vi "Check for Contained Data Type.vi"(4 "Type Specific Details":T1, 6 "Check VI Refnum Connector Pane? (F)":bool, 8 "error in (no error)":errorcluster, 10 "Data Type to Find":T2, 11 "Data Type":variant) -> (0 "error out":errorcluster, 2 "Contains Data Type to Find?":bool, 3 "dup Data Type":variant)   [LabVIEW 2020]
doc: "This VI is deprecated. Use the following VI instead:\n\nvi.lib\\Utility\\Data Type\\Check for Contained Data Type.vi\n\nThis VI checks the \"Data Type\" input to see if it contains any sub-types that are of type \"Data Type to Find\". If so, the \"Contains Data Type to Find?\" output is True.\n\nFor example, if \"Data Type\" is a cluster containing many items, including a Boolean data type, if \"Data Type to Find\" is \"Boolean\", the VI will return a \"Contains Data Type to Find?\" value of True."
uses:
  <vilib>/Utility/VariantDataType/Type.ctl
  <vilib>/Utility/VariantDataType/Type Specific Details.ctl
  <vilib>/Utility/VariantDataType/VariantType.lvlib
panel:
  # "This VI is deprecated. Use the following VI instead:\n\nvi.lib\\Utility\\Data Type\\Check for Contained Data Type.vi"
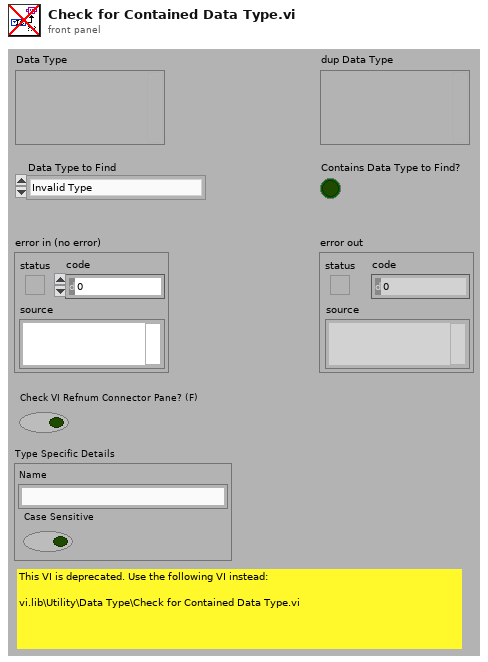
[diagram p1: front panel]
types:
  T1 = typedef "Type Specific Details.ctl" = cluster{"Name":string, "Case Sensitive":bool}
  T2 = typedef "VariantType.lvlib/Type.ctl" = enum8{"Invalid Type", "Void", "I8", "I16", "I32", "I64", "U8", "U16", "U32", "U64", "Single Float", "Double Float", "Extended Float", "Single Complex", "Double Complex", "Extended Complex", "Enum U8", "Enum U16", "Enum U32", "Enum U64", "Single Float With Unit", "Double Float With Unit", "Extended Float With Unit", "Single Complex with Unit", "Double Complex with Unit", "Extended Complex with Unit", "Boolean", "String", "Path", "Picture", "Tag", "Array", "Cluster", "Variant", "LV Variant", "Waveform", "Timestamp", "Digital Waveform", "Digital Data", "ExpressData", "Refnum", "External Data", "VI", "Poly VI", "LabVIEW Class Instance", "Fixed Point"}
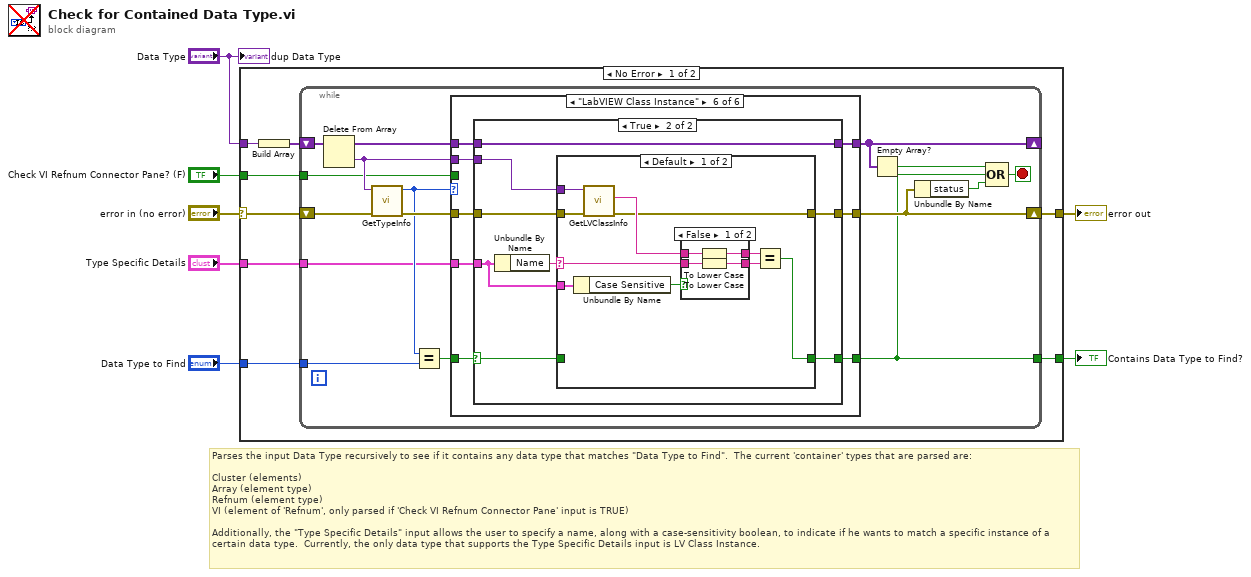
[diagram p0: block diagram]
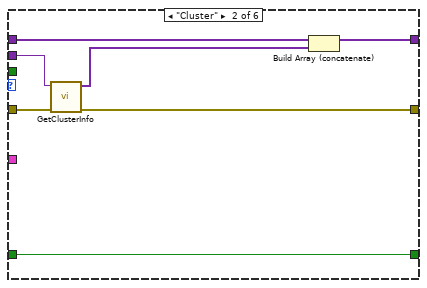
[diagram p3: hidden frame]
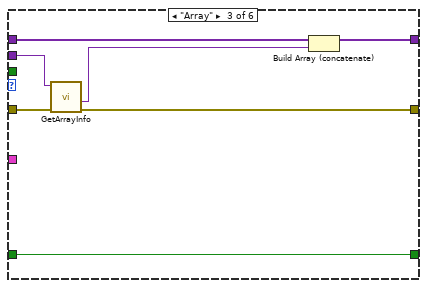
[diagram p4: hidden frame]
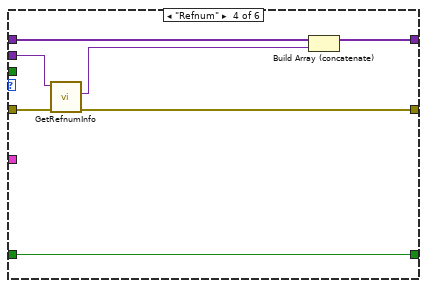
[diagram p5: hidden frame]
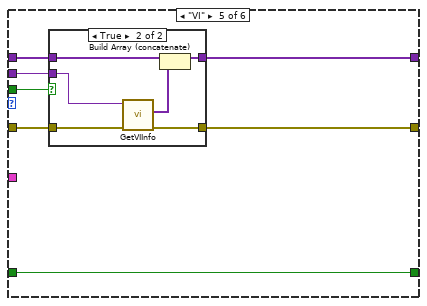
[diagram p6: hidden frame]
diagram:
  # "Parses the input Data Type recursively to see if it contains any data type that matches \"Data Type to Find\".  The current 'container' types that are parsed are:\n\nCluster (elements)\nArray (element type)\nRefnum (element type)\nVI (element of 'Refnum', only parsed if 'Check VI Refnum Connector Pane' input is TRUE)\n\nAdditionally, the \"Type Specific Details\" input allows the user to specify a name, along with a case-sensitivity boolean, to indicate if he wants to match a specific instance of a certain data type.  Currently, the only data type that supports the Type Specific Details input is LV Class Instance."
  n1 = case shown="No Error" "error in (no error)" {
    selector: "error in (no error)" -> [w12 w108]
    tunnel: "Data Type" -> [w15 _]
    tunnel: [w13 w108] -> w7
    tunnel: [w11 _] -> w5
    tunnel: "Data Type to Find" -> [w10 _]
    tunnel: "Check VI Refnum Connector Pane? (F)" -> [w9 _]
    tunnel: "Type Specific Details" -> [w8 _]
    frame No Error {
      n2 = Build Array(w15) -> (w14:variant[])
      n3 = while {
        shift-right: [w27] -> _
        shift-left: w14 -> [w31]
        shift-right: [w22] -> w13
        shift-left: w12 -> [w30]
        tunnel: [w16] -> w11
        tunnel: w10 -> [w20]
        tunnel: w9 -> [w19]
        tunnel: w8 -> [w18]
        stop <- w25 stop-if-true
        n4 = Delete From Array(array=w31) -> (deleted portion=w24:variant, array with subset deleted=w28:variant[])  [unwired: 2 in]
        n5 = call <vilib>:"GetTypeInfo.vi"("error in (no error)"=w30, "Variant"=w24) -> ("error out"=w29:errorcluster, "Type Enum"=w23:T2)  [unwired: 5 in, 3 out]
        n6 = Equal?(x=w23, y=w20) -> (x = y?=w17:bool)
        n7 = case shown="\"LabVIEW Class Instance\"" w23 {
          tunnel: w29 -> [w34 w41 w48 w55 w61 w78]
          tunnel: w28 -> [w33 w39 w45 w53 w59 w72]
          tunnel: [w33 w37 w44 w51 w58 w71] -> w27
          tunnel: [w34 w36 w46 w50 w60 w77] -> w22
          tunnel: w24 -> [_ w40 w47 w54 w57 w75]
          tunnel: w19 -> [_ _ _ _ w62 _]
          tunnel: w18 -> [_ _ _ _ _ w74]
          tunnel: w17 -> [w32 w35 w42 w49 w56 w73]
          tunnel: [w32 w35 w42 w49 w56 w76] -> w16
          frame Default {
          }
          frame "Cluster" {
            n8 = call <vilib>:"GetClusterInfo.vi"("error in (no error)"=w41, "Variant"=w40) -> ("error out"=w36:errorcluster, "Cluster Elements"=w38:variant[])  [unwired: 8 in]
            n9 = Build Array (concatenate)(w39, w38) -> (w37:variant[])
          }
          frame "Array" {
            n10 = call <vilib>:"GetArrayInfo.vi"("error in (no error)"=w48, "Variant"=w47) -> ("error out"=w46:errorcluster, "ArrayElement"=w43:variant)  [unwired: 6 in, 2 out]
            n11 = Build Array (concatenate)(w45, w43) -> (w44:variant[])
          }
          frame "Refnum" {
            n12 = call <vilib>:"GetRefnumInfo.vi"("error in (no error)"=w55, "Variant"=w54) -> ("error out"=w50:errorcluster, "StrictType"=w52:variant)  [unwired: 6 in, 2 out]
            n13 = Build Array (concatenate)(w53, w52) -> (w51:variant[])
          }
          frame "VI" {
            n14 = case shown="True" w62 {
              tunnel: w61 -> [w64 w70]
              tunnel: [w64 w69] -> w60
              tunnel: w59 -> [w63 w67]
              tunnel: [w63 w66] -> w58
              tunnel: w57 -> [_ w68]
              frame False {
              }
              frame True {
                n15 = call <vilib>:"GetVIInfo.vi"("error in (no error)"=w70, "Variant"=w68) -> ("error out"=w69:errorcluster, "VI Terminal Types"=w65:variant[])  [unwired: 5 in, 3 out]
                n16 = Build Array (concatenate)(w67, w65) -> (w66:variant[])
              }
            }
          }
          frame "LabVIEW Class Instance" {
            n17 = case shown="True" w73 {
              selector: w73 -> [w79 w83]
              tunnel: w78 -> [w80 w88]
              tunnel: [w80 w87] -> w77
              tunnel: [w79 w86] -> w76
              tunnel: w75 -> [_ w85]
              tunnel: w74 -> [_ w84]
              tunnel: w72 -> [w81 w82]
              tunnel: [w81 w82] -> w71
              frame False {
              }
              frame True {
                n18 = Unbundle By Name(w84) -> ("Name"=w89:string)
                n19 = case shown="Default" w89 {
                  selector: w89 -> [w95 _]
                  tunnel: w83 -> [_ w106]
                  tunnel: [w93 w107] -> w87
                  tunnel: w88 -> [w99 w107]
                  tunnel: [w90 w106] -> w86
                  tunnel: w85 -> [w98 _]
                  tunnel: w84 -> [w97 _]
                  frame Default {
                    n20 = Unbundle By Name(w97) -> ("Case Sensitive"=w96:bool)
                    n21 = call <vilib>:"GetLVClassInfo.vi"("error in (no error)"=w99, "Variant"=w98) -> ("error out"=w93:errorcluster, "LV Class File Name"=w94:string)  [unwired: 7 in, 1 out]
                    n22 = case shown="False" w96 {
                      tunnel: w95 -> [w103 w105]
                      tunnel: [w102 w105] -> w91
                      tunnel: w94 -> [w101 w104]
                      tunnel: [w100 w104] -> w92
                      frame False {
                        n23 = To Lower Case(string=w101) -> (all lower case string=w100:string)
                        n24 = To Lower Case(string=w103) -> (all lower case string=w102:string)
                      }
                      frame True {
                      }
                    }
                    n25 = Equal?(x=w92, y=w91) -> (x = y?=w90:bool)
                  }
                  frame "" {
                  }
                }
              }
            }
          }
        }
        n26 = Empty Array?(array=w27) -> (empty?=w26:bool)
        n27 = Unbundle By Name(w22) -> ("status"=w21:bool)
        n28 = Compound Arithmetic op=OR(w26, w16, w21) -> (w25:bool)
      }
    }
    frame Error {
    }
  }
  "Contains Data Type to Find?" <- w5
  "error out" <- w7
  "dup Data Type" <- "Data Type"
